vi "XLP80_CAN_MaskBytesMotorola.vi"(8 "Length":i32=16, 9 "StartBit":i32=27, 10 "Input":bool[](array[boolean])=[FALSE, FALSE, TRUE, FALSE, FALSE, TRUE, TRUE, FALSE, FALSE, FALSE, FALSE, FALSE, FALSE, FALSE, FALSE, FALSE], 11 "ID IN":bool[](array[boolean])) -> (3 "ID OUT":bool[](array[boolean]))   [LabVIEW 2021]
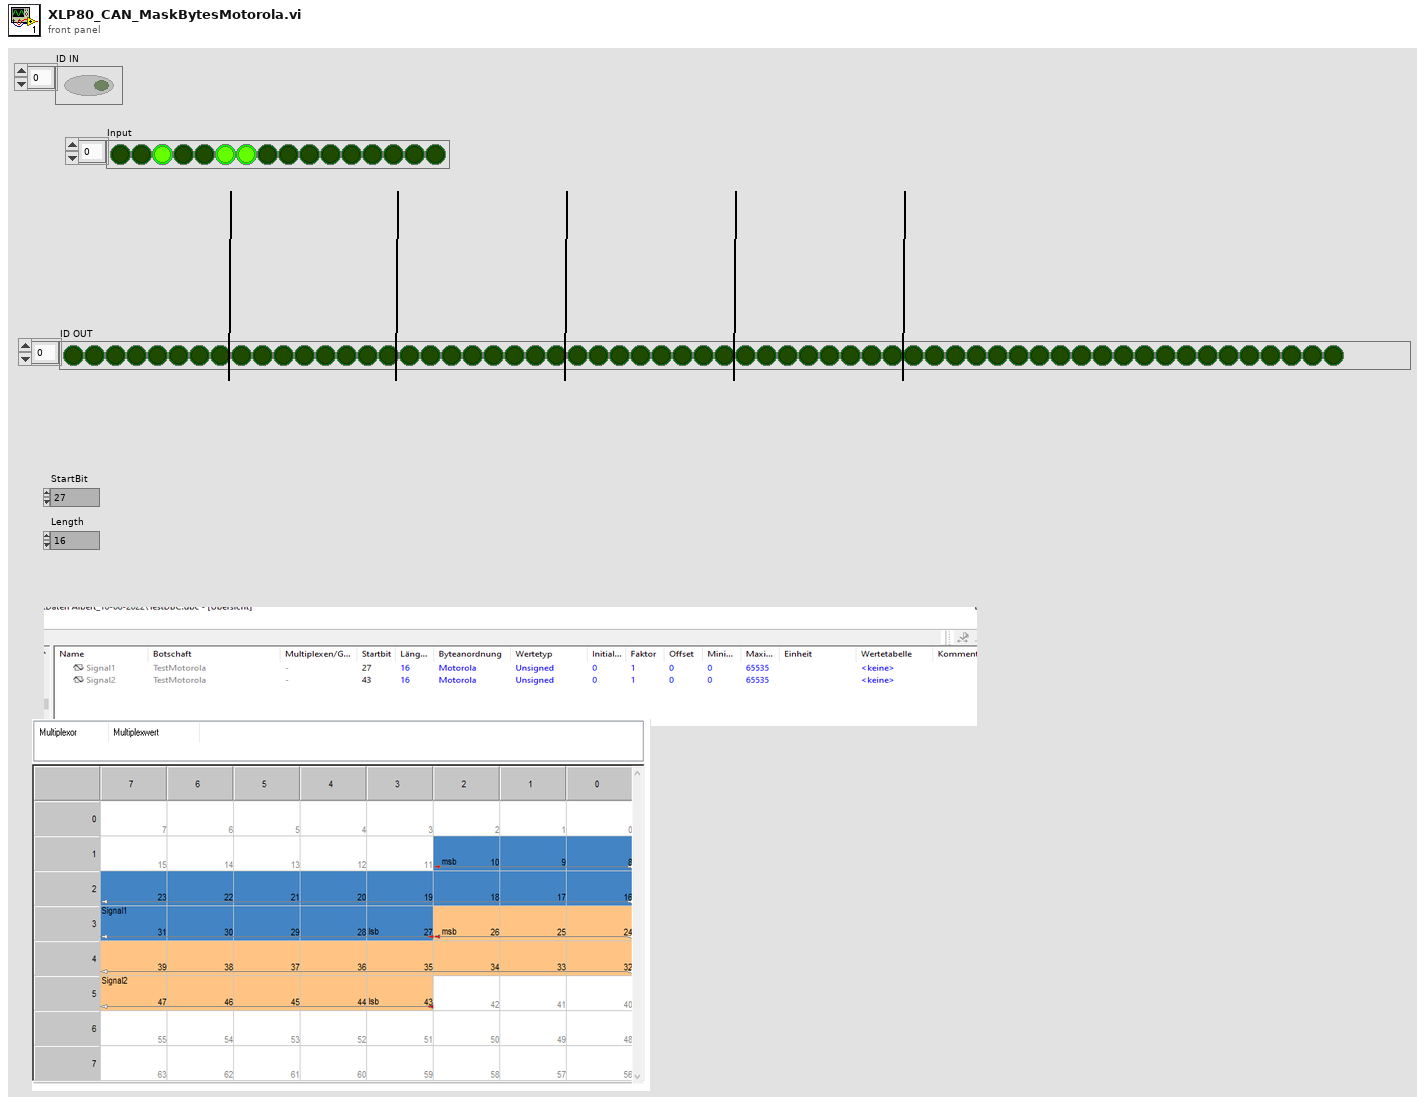
[diagram p1: front panel]
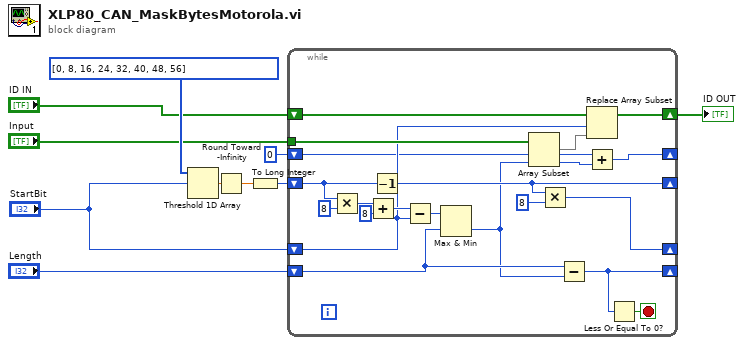
[diagram p0: block diagram]
diagram:
  n1 = Threshold 1D Array(2:"StartBit", 3:i32[] [0, 8, 16, 24, 32, 40, 48, 56] ("Array")) -> (0:w9:dbl)  [unwired: 1 in]
  n2 = Round Toward -Infinity(1:w9) -> (0:w8:dbl)
  n3 = To Long Integer(number=w8) -> (32bit integer=w4:i32)
  n4 = while {
    shift-right: [w14] -> w3
    shift-left: "ID IN" -> [w30]
    tunnel: "Input" -> [w29]
    shift-right: [w11] -> _
    shift-left: 0 ("index") -> [w13]
    shift-right: [w28] -> _
    shift-left: "Length" -> [w22]
    shift-right: [w18] -> _
    shift-left: w4 -> [w19]
    shift-right: [w16] -> _
    shift-left: "StartBit" -> [w15]
    stop <- w20 stop-if-true
    n5 = Multiply(x=w19, y=8) -> (x*y=w24:i32)
    n6 = Add(x=w24, y=8) -> (x+y=w26:i32)
    n7 = Decrement(x=w19) -> (x-1=w18:i32)
    n8 = Subtract(x=w26, y=w15) -> (x-y=w27:i32)
    n9 = Max & Min(x=w27, y=w22) -> (min(x,y)=w12:i32)  [unwired: 1 out]
    n10 = Array Subset(array=w29, index=w13, length=w12) -> (w21:bool[])
    n11 = Multiply(x=w18, y=8) -> (x*y=w16:i32)
    n12 = Subtract(x=w22, y=w12) -> (x-y=w28:i32)
    n13 = Replace Array Subset(array=w30, new element=w21, index=w15) -> (w14:bool[])
    n14 = Add(x=w13, y=w12) -> (x+y=w11:i32)
    n15 = Less Or Equal To 0?(x=w28) -> (x <= 0?=w20:bool)
  }
  "ID OUT" <- w3
